vi "video.get.vi"(8 "error in":errorcluster, 10 "videoRid":string, 11 "Nominal Client in":refnum<class "Nominal Client.lvclass">) -> (0 "error out":errorcluster, 2 "Pretty JSON Out":string, 3 "Nominal Client out":refnum<class "Nominal Client.lvclass">)   [LabVIEW 2018, in "Nominal Client.lvclass"]
doc: "Returns video metadata associated with a video rid."
uses:
  Nominal Client.lvclass
  Nominal Client.lvclass/Nominal Client.ctl
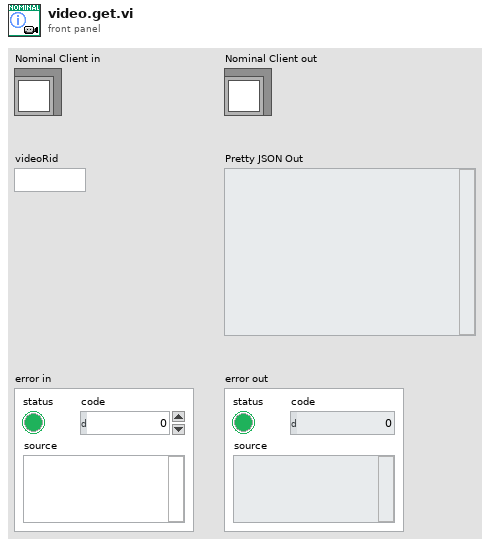
[diagram p1: front panel]
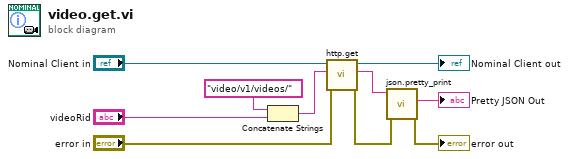
[diagram p0: block diagram]
diagram:
  n1 = Concatenate Strings("video/v1/videos/" ("Path"), "videoRid") -> (w5:string)
  n2 = call "http.get.vi"("error in"="error in", "Path"=w5, "Nominal Client in"="Nominal Client in") -> ("error out"=w2:errorcluster, "Response"=w4:string, "Nominal Client out"=→"Nominal Client out":refnum<class "Nominal Client.lvclass">)  [unwired: 5 in, 1 out]
  n3 = call "json.pretty_print.vi"("error in"=w2, "JSON in"=w4) -> ("error out"=→"error out":errorcluster, "Pretty JSON Out"=→"Pretty JSON Out":string)  [unwired: 8 in]
